vi "Generate_WayPoints_Hopping_Light.vi"(11 "Input Cluster":T2={"Scan Rate (um/s)"=15.0, "X Start"=15.0, "X End"=15.0, "Y Start"=15.0, "Y End"=15.0, " Z Start"=15.0, "HoppingDistance"=1.0, "V"=15.0, "Z End"=15.0, "Approach Rate Hopping (um/s)"=15.0, "Retract Rate (um/s)"=15.0, "V 2"=15.0, "Approach Rate (um/s)"=15.0, "Hold_Time"=1.0}) -> (0 "output cluster":T1)   [LabVIEW 2023]
uses:
  TypeDefs/WayPointCluster.ctl
  User_Vi/Settings.vi
panel:
  in  "WayPointCluster":T1
  out "Y  P":dbl
  out "X  P":dbl
  out "HoppingDistanceX":dbl
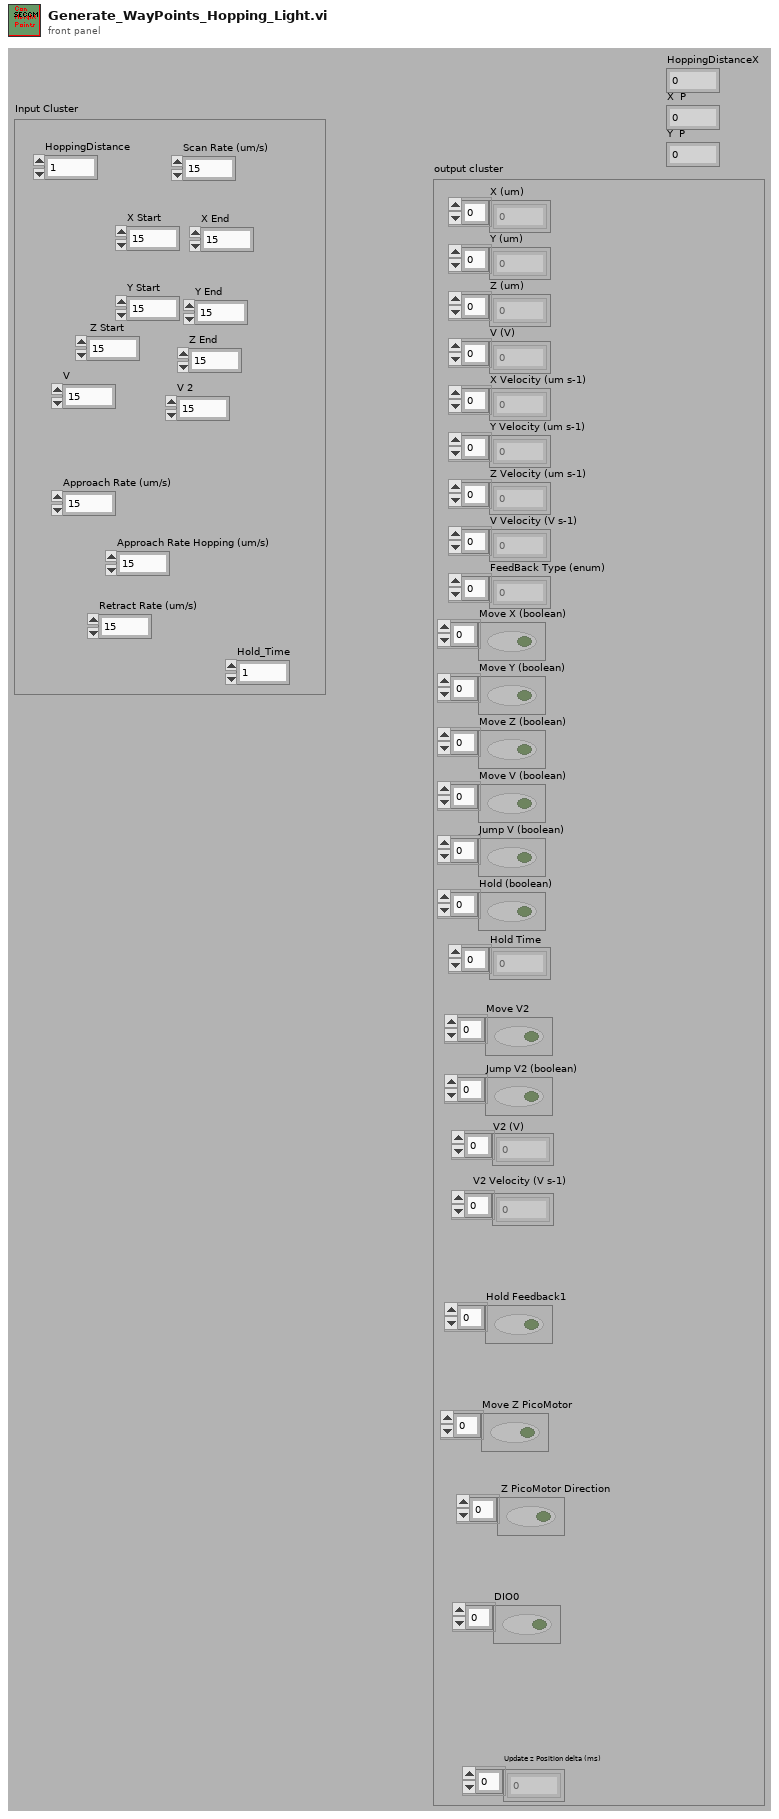
[diagram p1: front panel]
types:
  T1 = typedef "WayPointCluster.ctl" = cluster{"X (um)":dbl[], "Y (um)":dbl[], "Z (um)":dbl[], "V (V)":dbl[], "X Velocity (um s-1)":dbl[], "Y Velocity (um s-1)":dbl[], "Z Velocity (um s-1)":dbl[], "V Velocity (V s-1)":dbl[], "FeedBack Type (enum)":u16[], "Move X (boolean)":bool[], "Move Y (boolean)":bool[], "Move Z (boolean)":bool[], "Move V (boolean)":bool[], "Jump V (boolean)":bool[], "Hold (boolean)":bool[], "Hold Time":u32[], "V2 (V)":dbl[], "Move V2":bool[], "V2 Velocity (V s-1)":dbl[], "Jump V2 (boolean)":bool[], "Update z Position delta (ms)":i16[], "Hold Feedback1":bool[], "Move Z PicoMotor":bool[], " Z PicoMotor Direction":bool[], "DIO0":bool[]}
  T2 = cluster{"Scan Rate (um/s)":dbl, "X Start":dbl, "X End":dbl, "Y Start":dbl, "Y End":dbl, " Z Start":dbl, "HoppingDistance":dbl, "V":dbl, "Z End":dbl, "Approach Rate Hopping (um/s)":dbl, "Retract Rate (um/s)":dbl, "V 2":dbl, "Approach Rate (um/s)":dbl, "Hold_Time":dbl}
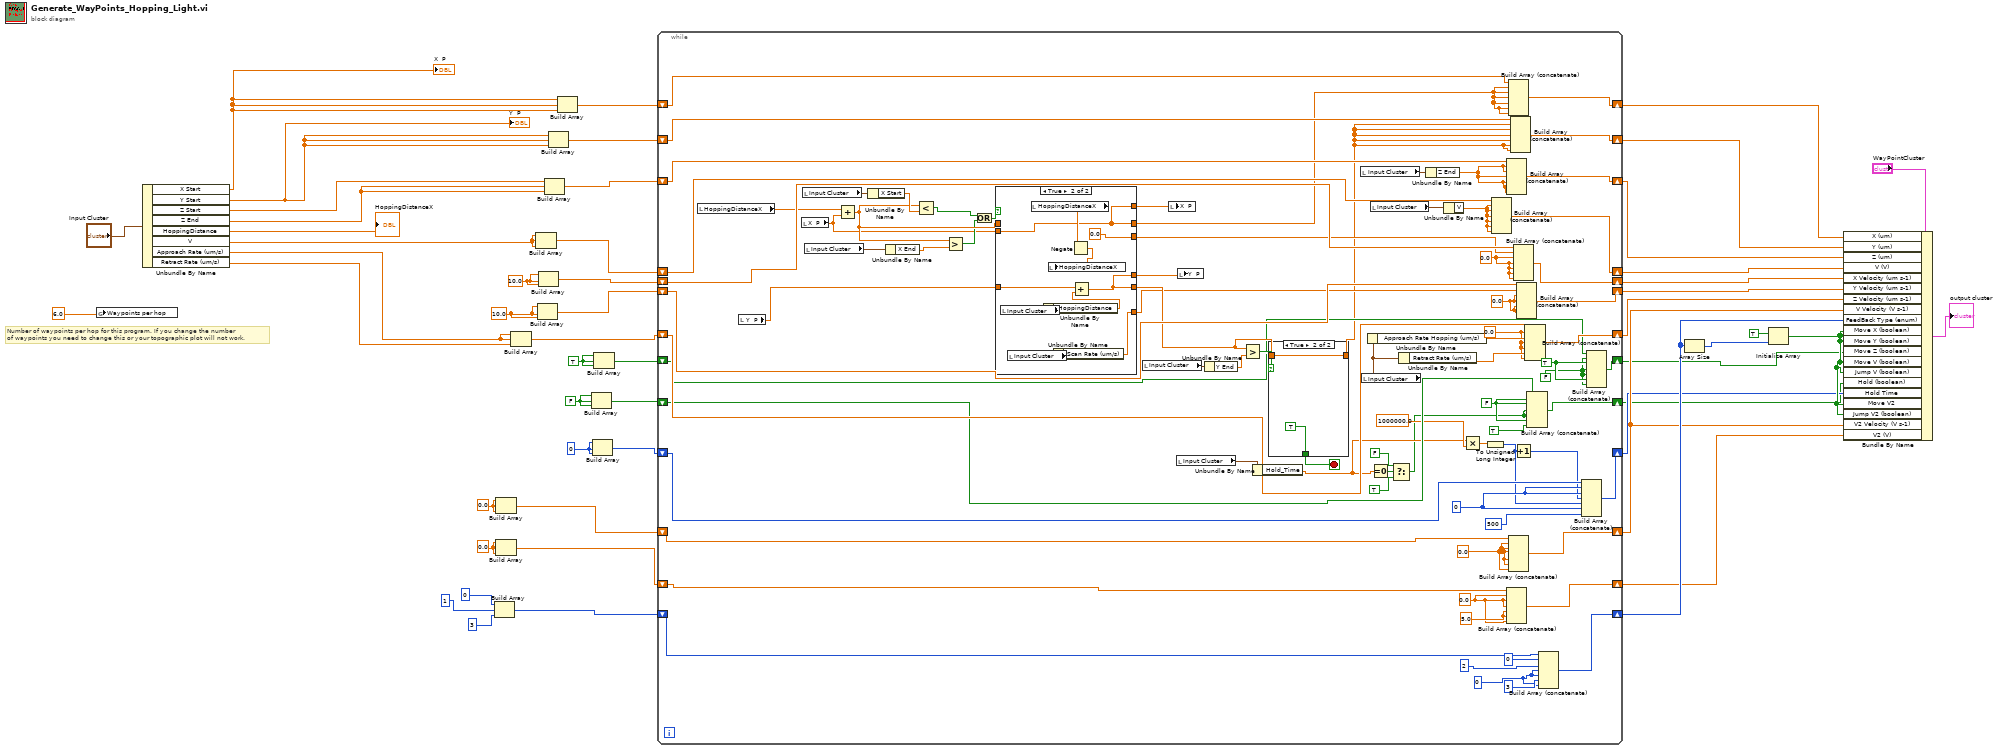
[diagram p0: block diagram]
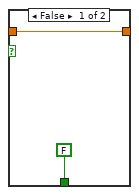
[diagram p2: hidden frame]
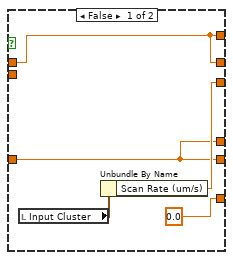
[diagram p3: hidden frame]
diagram:
  w3 = TRUE
  w8 = u16 0 ("element")
  w9 = FALSE
  w14 = 0.0 ("element")
  w23 = 10.0 ("element")
  w22 = 10.0 ("element")
  w20 = 0.0 ("element")
  # "Number of waypoints per hop for this program. If you change the number\nof waypoints you need to change this or your topographic plot will not work."
  n1 = global write "Settings.vi" "Waypoints per hop"(6.0) -> ()
  n2 = Unbundle By Name("Input Cluster") -> ("X Start"=w35:dbl, "Y Start"=w29:dbl, "Z Start"=w28:dbl, "Z End"=w25:dbl, "HoppingDistance"=→"HoppingDistanceX":dbl, "V"=w26:dbl, "Approach Rate (um/s)"=w21:dbl, "Retract Rate (um/s)"=w34:dbl)
  "X  P" <- w35
  "Y  P" <- w29
  n3 = Build Array(u16 0 ("element"), u16 1 ("element"), u16 3 ("element")) -> (w36:u16[])
  n4 = Build Array(w20, w20, w20) -> (w37:dbl[])
  n5 = Build Array(w14, w14, w14) -> (w13:dbl[])
  n6 = Build Array(w21, w21, w34) -> (w39:dbl[])
  n7 = Build Array(w26, w26, w26) -> (w44:dbl[])
  n8 = Build Array(w22, w22, w22) -> (w41:dbl[])
  n9 = Build Array(w23, w23, w23) -> (w42:dbl[])
  n10 = Build Array(w28, w25, w25) -> (w46:dbl[])
  n11 = Build Array(w29, w29, w29) -> (w47:dbl[])
  n12 = Build Array(w35, w35, w35) -> (w49:dbl[])
  n13 = Build Array(w9, w9, w9) -> (w10:bool[])
  n14 = Build Array(w8, w8, w8) -> (w11:u16[])
  n15 = Build Array(w3, w3, w3) -> (w2:bool[])
  n16 = while {
    shift-right: [w129] -> w48
    shift-left: w49 -> [w130]
    shift-right: [w121] -> w30
    shift-left: w47 -> [w111]
    shift-right: [w120] -> w45
    shift-left: w46 -> [w128]
    shift-right: [w119] -> w43
    shift-left: w44 -> [w127]
    shift-right: [w118] -> w31
    shift-left: w42 -> [w126]
    shift-right: [w117] -> w40
    shift-left: w41 -> [w125]
    shift-right: [w116] -> w38
    shift-left: w39 -> [w124]
    shift-right: [w115] -> w15
    shift-left: w37 -> [w123]
    shift-right: [w114] -> w27
    shift-left: w36 -> [w122]
    shift-right: [w89] -> w12
    shift-left: w13 -> [w88]
    shift-right: [w85] -> w7
    shift-left: w11 -> [w81]
    shift-right: [w86] -> w5
    shift-left: w10 -> [w82]
    shift-right: [w71] -> w4
    shift-left: w2 -> [w70]
    stop <- w101 stop-if-true
    w58 = FALSE
    w72 = TRUE
    w52 = u32 0 ("element")
    w83 = u32 0 ("element")
    w84 = FALSE
    w87 = 5.0 ("element")
    w53 = 0.0 ("element")
    w60 = 0.0 ("element")
    w61 = 0.0 ("element")
    w54 = 0.0 ("element")
    w59 = 0.0 ("element")
    n17 = local read "HoppingDistanceX"() -> (w90:dbl)
    n18 = local read "Y  P"() -> (w99:dbl)
    n19 = local read "X  P"() -> (w91:dbl)
    n20 = local read "Input Cluster"() -> (w132:T2)
    n21 = local read "Input Cluster"() -> (w131:T2)
    n22 = Add(x=w90, y=w91) -> (x+y=w107:dbl)
    n23 = Unbundle By Name(w132) -> ("X Start"=w110:dbl)
    n24 = Unbundle By Name(w131) -> ("X End"=w108:dbl)
    n25 = Less?(x=w107, y=w110) -> (x < y?=w109:bool)
    n26 = Greater?(x=w107, y=w108) -> (0:w106:bool)
    n27 = Or(x=w109, y=w106) -> (x .or. y?=w105:bool)
    n28 = case shown="True" w105 {
      tunnel: w107 -> [w137 _]
      tunnel: [w137 w143] -> w65
      tunnel: w91 -> [_ w143]
      tunnel: w99 -> [w138 w144]
      tunnel: [w138 w142] -> w98
      tunnel: [w140 0.0] -> w93
      tunnel: [0.0 w145] -> w92
      tunnel: [w138 w142] -> w97
      tunnel: [w137 w143] -> w96
      frame False {
        n29 = local read "Input Cluster"() -> (w141:T2)
        n30 = Unbundle By Name(w141) -> ("Scan Rate (um/s)"=w140:dbl)
      }
      frame True {
        n31 = local read "Input Cluster"() -> (w149:T2)
        n32 = local read "Input Cluster"() -> (w147:T2)
        n33 = local read "HoppingDistanceX"() -> (w151:dbl)
        n34 = Unbundle By Name(w149) -> ("HoppingDistance"=w148:dbl)
        n35 = Unbundle By Name(w147) -> ("Scan Rate (um/s)"=w145:dbl)
        n36 = Negate(x=w151) -> (-x=w150:dbl)
        n37 = local write "HoppingDistanceX"(w150) -> ()
        n38 = Add(x=w144, y=w148) -> (x+y=w142:dbl)
      }
    }
    n39 = local read "Input Cluster"() -> (w104:T2)
    n40 = local write "X  P"(w96) -> ()
    n41 = local read "Input Cluster"() -> (w76:T2)
    n42 = local write "Y  P"(w97) -> ()
    n43 = Unbundle By Name(w104) -> ("Y End"=w103:dbl)
    n44 = Greater?(x=w98, y=w103) -> (0:w102:bool)
    n45 = Unbundle By Name(w76) -> ("Hold_Time"=w66:dbl)
    n46 = case shown="True" w102 {
      tunnel: w98 -> [w134 w136]
      tunnel: [w134 w136] -> w64
      tunnel: [FALSE TRUE] -> w101
      frame False {
      }
      frame True {
      }
    }
    n47 = local read "Input Cluster"() -> (w113:T2)
    n48 = local read "Input Cluster"() -> (w100:T2)
    n49 = Unbundle By Name(w100) -> ("Approach Rate Hopping (um/s)"=w94:dbl)
    n50 = local read "Input Cluster"() -> (w112:T2)
    n51 = Equal To 0?(x=w66) -> (x = 0?=w69:bool)
    n52 = Select(t=FALSE, s=w69, f=TRUE) -> (s? t:f=w57:bool)
    n53 = Unbundle By Name(w100) -> ("Retract Rate (um/s)"=w80:dbl)
    n54 = Unbundle By Name(w113) -> ("Z End"=w63:dbl)
    n55 = Unbundle By Name(w112) -> ("V"=w62:dbl)
    n56 = Multiply(x=w66, y=1000000.0 ("element")) -> (x*y=w79:dbl)
    n57 = To Unsigned Long Integer(number=w79) -> (unsigned 32bit integer=w77:u32)
    n58 = Build Array (concatenate)(w127, w62, w62, w62, w62, w62, w62) -> (w119:dbl[])
    n59 = Build Array (concatenate)(w128, w63, w63, w63, w63, w63, w63) -> (w120:dbl[])
    n60 = Build Array (concatenate)(w88, w53, w53, w53, w87, w87, w53) -> (w89:dbl[])
    n61 = Build Array (concatenate)(w130, w65, w65, w65, w65, w65, w65) -> (w129:dbl[])
    n62 = Build Array (concatenate)(w123, w54, w54, w54, w54, w54, w54) -> (w115:dbl[])
    n63 = Build Array (concatenate)(w111, w64, w64, w64, w64, w64, w64) -> (w121:dbl[])
    n64 = Build Array (concatenate)(w126, w93, w61, w61, w61, w61, w61) -> (w118:dbl[])
    n65 = Increment(x=w77) -> (x+1=w78:u32)
    n66 = Build Array (concatenate)(w125, w92, w60, w60, w60, w60, w60) -> (w117:dbl[])
    n67 = Build Array (concatenate)(w124, w59, w94, w59, w59, w80, w59) -> (w116:dbl[])
    n68 = Build Array (concatenate)(w82, w84, w84, w57, w57, w84, TRUE) -> (w86:bool[])
    n69 = Build Array (concatenate)(w122, u16 0 ("element"), u16 2 ("element"), w52, w52, u16 3 ("element"), w52) -> (w114:u32[])
    n70 = Build Array (concatenate)(w81, w83, w83, w78, w77, w83, u32 500 ("element")) -> (w85:u32[])
    n71 = Build Array (concatenate)(w70, w58, w72, w58, w58, w72, w58) -> (w71:bool[])
  }
  n72 = Array Size(array=w27) -> (size(s)=w32:i32)
  n73 = Initialize Array(TRUE, w32) -> (w16:bool[])
  n74 = Bundle By Name(cluster="WayPointCluster", "X (um)"=w48, "Y (um)"=w30, "Z (um)"=w45, "V (V)"=w43, "X Velocity (um s-1)"=w31, "Y Velocity (um s-1)"=w40, "Z Velocity (um s-1)"=w38, "V Velocity (V s-1)"=w15, "FeedBack Type (enum)"=w27, "Move X (boolean)"=w16, "Move Y (boolean)"=w16, "Move Z (boolean)"=w4, "Move V (boolean)"=w16, "Jump V (boolean)"=w16, "Hold (boolean)"=w5, "Hold Time"=w7, "Move V2"=w16, "Jump V2 (boolean)"=w16, "V2 Velocity (V s-1)"=w15, "V2 (V)"=w12) -> (→"output cluster":T1)
